vi "Close TLCamera.vi"(8 "error in (no error)":errorcluster, 11 "TLCamera reference":refnum<k24>) -> (0 "error out":errorcluster)   [LabVIEW 2015]
uses:
  C:/code/Host/Installer/Scientific Camera Interfaces/LabVIEW/64_bit/Library_X64/Thorlabs.TSI.TLCameraInterfaces.dll
  code/Host/Installer/Scientific Camera Interfaces/LabVIEW/64_bit/Library_X64/Thorlabs.TSI.TLCameraInterfaces.dll
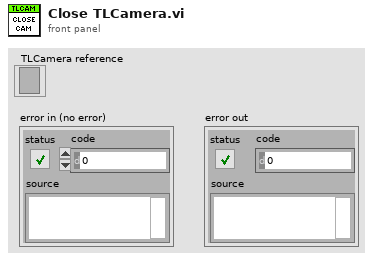
[diagram p1: front panel]
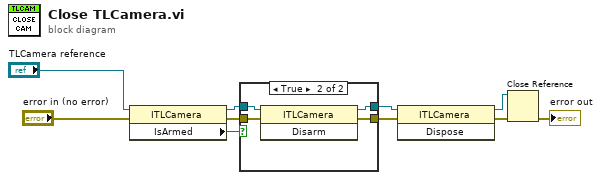
[diagram p0: block diagram]
diagram:
  n1 = property class="ITLCamera"(reference="TLCamera reference", error in="error in (no error)") -> (reference out=w3:refnum<k24>, error out=w5:errorcluster, "IsArmed"=w2:bool)
  n2 = case shown="True" w2 {
    tunnel: w3 -> [w12 w16]
    tunnel: w5 -> [w11 w15]
    tunnel: [w12 w14] -> w6
    tunnel: [w11 w13] -> w7
    frame False {
    }
    frame True {
      n3 = invoke class="ITLCamera" method="Disarm"(reference=w16, error in=w15) -> (reference out=w14:refnum<k24>, error out=w13:errorcluster)  [unwired: 1 in, 1 out]
    }
  }
  n4 = invoke class="ITLCamera" method="Dispose"(reference=w6, error in=w7) -> (reference out=w9:refnum<k24>, error out=w8:errorcluster)  [unwired: 1 in, 1 out]
  n5 = Close Reference(reference=w9, error in (no error)=w8) -> (error out=→"error out":errorcluster)
